vi "Attocubes_test.vi"() -> ()   [LabVIEW 2019]
panel:
  in  "Stop":bool
  out "Position [µm | m°] 2":dbl format="%.3g"
  in  "Axis IN":u8(ring) items=["1", "2", "3"]
  out "axis out":u8(ring) items=["1", "2", "3"]
  out "Position [µm | m°]":dbl format="%.3g"
  out "*(type *) &x":u8
  out "Numeric":u8
  out "PosZ":dbl
  out "PosY":dbl
  out "PosX":dbl
  out "DCLvlZ":dbl
  out "FreqZ":dbl
  out "AmpZ":dbl
  out "DCLvlY":dbl
  out "FreqY":dbl
  out "AmpY":dbl
  out "DCLvlX":dbl
  out "FreqX":dbl
  out "AmpX":dbl
  out "additional features":T1
  out "features":u32 format="%08b"
  out "error ANC350v4_Dis/Connect 2":errorcluster
  out "error ANC350v4_discover":errorcluster
  out "output cluster":T2 {"DeviceType" items=["ANC350res", "ANC350num", "ANC350fps", "No device / invalid"]; "ID" format="%x"}
  out "error ANC350v4_Dis/Connect":errorcluster
  out "ANC350v4 found":u32
  out "ANC350_Handle":u64
  out "ourDLL":path
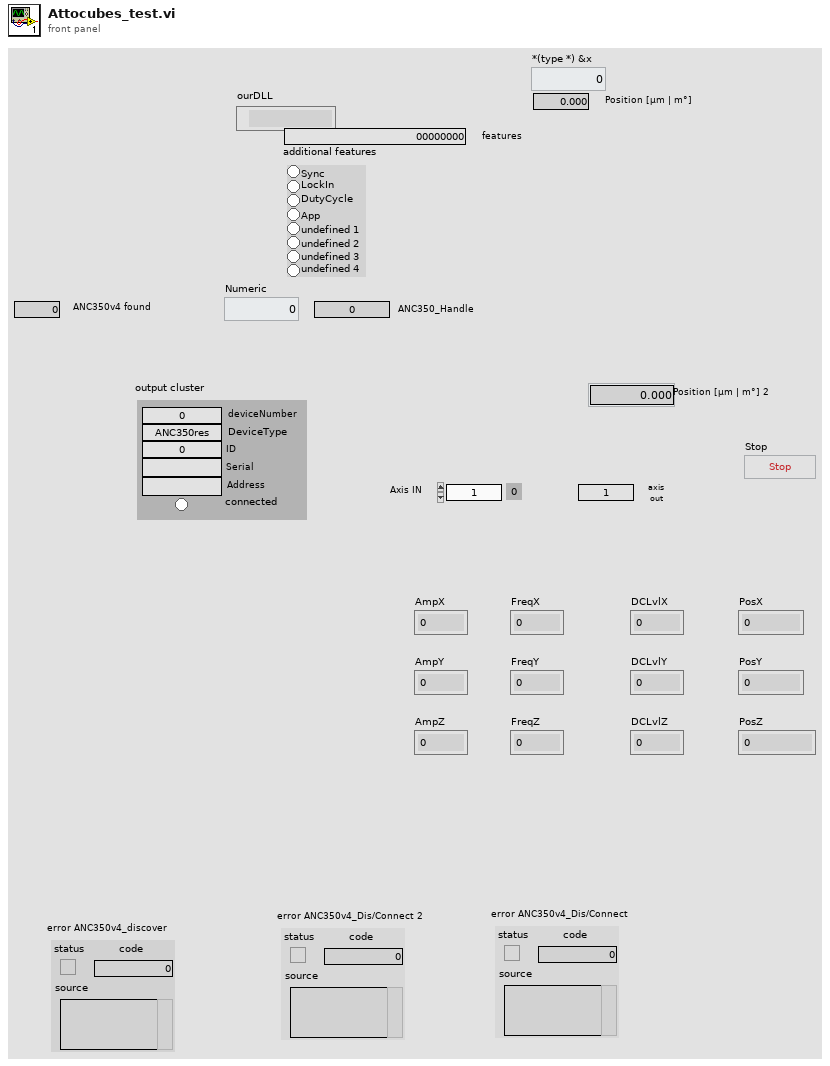
[diagram p1: front panel]
types:
  T1 = cluster{"Sync":bool, "LockIn":bool, "DutyCycle":bool, "App":bool, "undefined 1":bool, "undefined 2":bool, "undefined 3":bool, "undefined 4":bool, "undefined 7":bool}
  T2 = cluster{"deviceNumber":i32, "DeviceType":i32, "ID":u32, "Serial":string, "Address":string, "connected":bool}
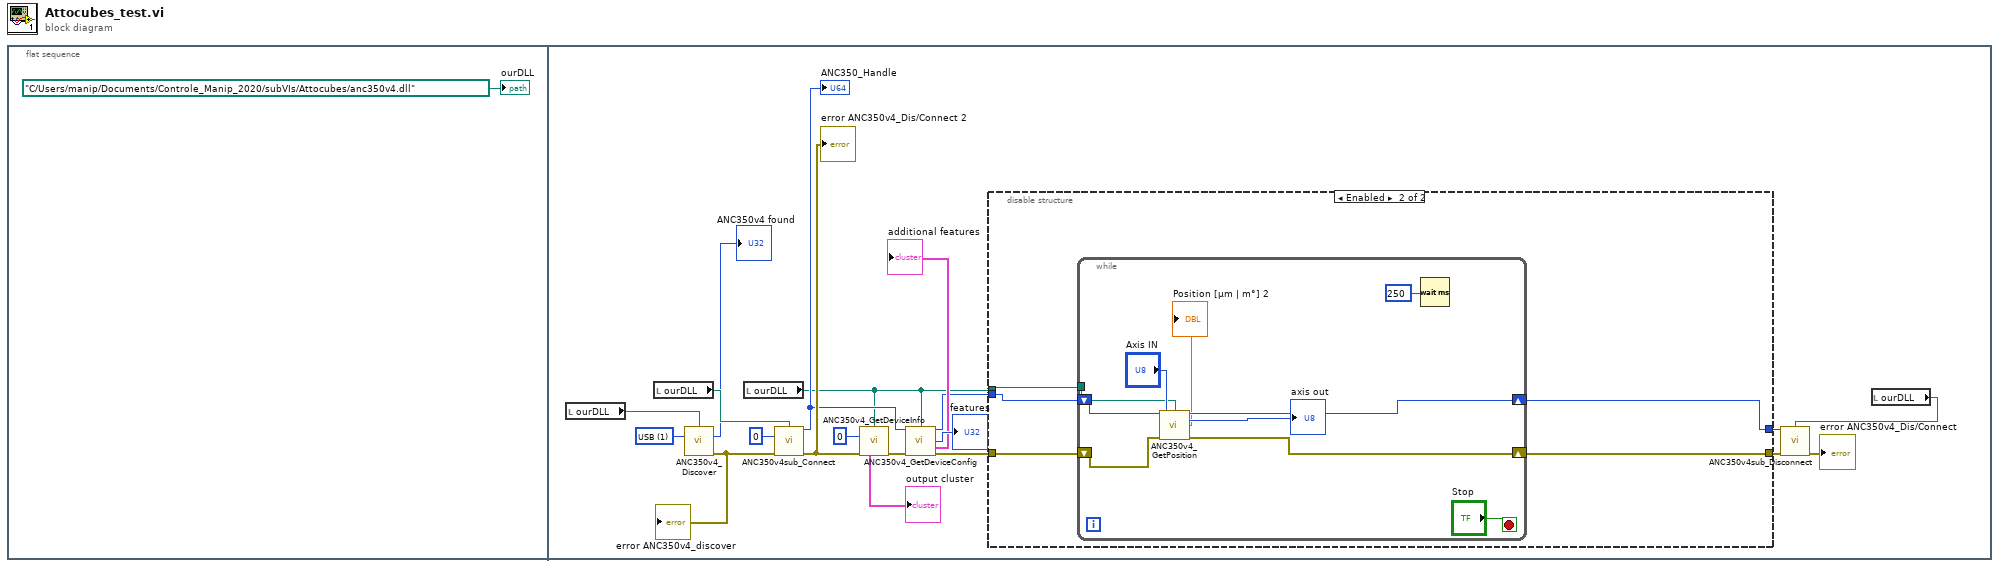
[diagram p0: block diagram]
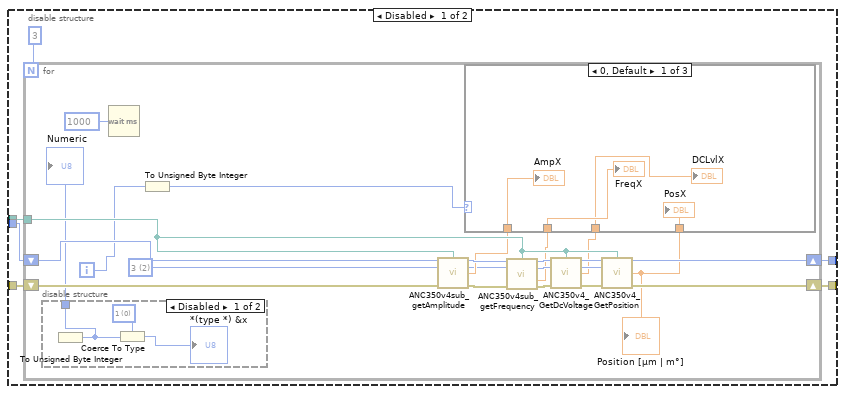
[diagram p2: hidden frame]
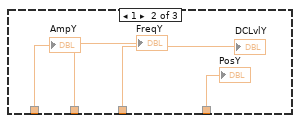
[diagram p4: hidden frame]
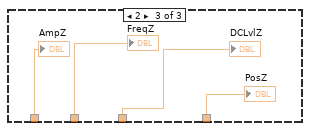
[diagram p5: hidden frame]
diagram:
  n1 = flat-sequence {
    frame #0 {
      "ourDLL" <- path "C:/Users/manip/Documents/Controle_Manip_2020/subVIs/Attocubes/anc350v4.dll"
    }
    frame #1 {
      w21 = u32 1 items=["None", "USB", "TCP", "All"] ("Interface types")
      n2 = local read "ourDLL"() -> (w14:path)
      n3 = local read "ourDLL"() -> (w20:path)
      n4 = call "ANC350v4_Discover.vi"("Path to *.DLL"=w14, "Interface types"=w21) -> ("ANC350v4 found"=→"ANC350v4 found":u32, "error ANC350v4_discover"=w19:errorcluster)  [unwired: 12 in]
      "error ANC350v4_discover" <- w19
      n5 = local read "ourDLL"() -> (w7:path)
      n6 = call "ANC350v4sub_Connect.vi"("Path to *.DLL"=w20, "deviceNumber"=0, "error in"=w19) -> ("ANC350v4_Handle_Out"=w11:u64, "error ANC350v4_Dis/Connect"=w15:errorcluster)  [unwired: 11 in]
      "ANC350_Handle" <- w11
      "error ANC350v4_Dis/Connect 2" <- w15
      n7 = call "ANC350v4_GetDeviceInfo.vi"("Path to *.DLL"=w7, "deviceNumber"=u32 0, "error in"=w15) -> ("output cluster"=→"output cluster":T2, "Error_ANC350v4_getDeviceInfo"=w10:errorcluster)  [unwired: 5 in, 6 out]
      n8 = call "ANC350v4_GetDeviceConfig.vi"("deviceHandle"=w11, "Path to *.DLL"=w7, "error in"=w10) -> ("deviceHandle"=w6:u64, "features"=→"features":u32, "additional features"=→"additional features":T1, "Error_ANC350v4_getDeviceConfig"=w4:errorcluster)  [unwired: 9 in]
      n9 = disable-structure shown="Enabled" {
        disable-tunnel: w7 -> [w27 w66]
        disable-tunnel: w6 -> [w26 w70]
        disable-tunnel: [w25 w68] -> w5
        disable-tunnel: w4 -> [w24 w69]
        disable-tunnel: [w23 w67] -> w3
        frame Disabled {
          n10 = for {
            N: 3 -> [_]
            tunnel: w27 -> [w42]
            shift-right: [w40] -> w25
            shift-left: w24 -> [w39]
            shift-right: [w38] -> w23
            shift-left: w26 -> [w41]
            i -> [w29]
            w28 = u8 2 items=["1", "2", "3"] ("axis")
            n11 = disable-structure shown="Disabled" {
              disable-tunnel: [w51 _] -> w31
              frame Disabled {
                w53 = u8 0 items=["1", "2", "3"] ("axis")
                n12 = To Unsigned Byte Integer() -> (unsigned 8bit integer=w51:u8)  [unwired: 1 in]
                n13 = Coerce To Type(0:w51, 1:w53) -> (2:→"*(type *) &x":u8)
              }
              frame Enabled {
              }
            }
            "Numeric" <- w31
            n14 = Wait (ms)(milliseconds to wait=u32 1000) -> ()  [unwired: 1 out]
            n15 = To Unsigned Byte Integer(number=w29) -> (unsigned 8bit integer=w30:u8)
            n16 = call "ANC350v4sub_getAmplitude.vi"("deviceHandle"=w41, "Path to *.DLL"=w42, "axis"=w28, "error in"=w39) -> ("deviceHandle"=w43:u64, "axis"=w32:u8, "amplitude out"=w37:dbl, "error ANC350v4_Amplitude"=w44:errorcluster)  [unwired: 8 in]
            n17 = call "ANC350v4sub_getFrequency.vi"("deviceHandle"=w43, "Path to *.DLL"=w42, "axis"=w32, "error in"=w44) -> ("deviceHandle"=w47:u64, "axis"=w46:u8, "Frequency [Hz] out"=w36:dbl, "error ANC350v4_frequency"=w45:errorcluster)  [unwired: 8 in]
            n18 = call "ANC350v4_GetDcVoltage.vi"("deviceHandle"=w47, "Path to *.DLL"=w42, "axis"=w46, "error in"=w45) -> ("deviceHandle"=w50:u64, "axis"=w49:u8, "voltage"=w35:dbl, "error ANC350v4_getDcVoltage"=w48:errorcluster)  [unwired: 8 in]
            n19 = call "ANC350v4_GetPosition.vi"("deviceHandle"=w50, "Path to *.DLL"=w42, "axis"=w49, "error in"=w48) -> ("deviceHandle"=w38:u64, "Position [µm | m°]"=w34:dbl, "error ANC350v4_getPosition"=w40:errorcluster)  [unwired: 8 in, 1 out]
            "Position [µm | m°]" <- w34
            n20 = case shown="0, Default" w30 {
              tunnel: w37 -> [w57 w61 w65]
              tunnel: w36 -> [w56 w60 w64]
              tunnel: w35 -> [w55 w59 w63]
              tunnel: w34 -> [w54 w58 w62]
              frame 0, Default {
                "FreqX" <- w56
                "AmpX" <- w57
                "DCLvlX" <- w55
                "PosX" <- w54
              }
              frame 1 {
                "FreqY" <- w60
                "DCLvlY" <- w59
                "AmpY" <- w61
                "PosY" <- w58
              }
              frame 2 {
                "FreqZ" <- w64
                "DCLvlZ" <- w63
                "AmpZ" <- w65
                "PosZ" <- w62
              }
            }
          }
        }
        frame Enabled {
          n21 = while {
            tunnel: w66 -> [w74]
            shift-right: [w77] -> w67
            shift-left: w70 -> [w80]
            shift-right: [w78] -> w68
            shift-left: w69 -> [w79]
            stop <- "Stop" stop-if-true
            n22 = call "ANC350v4_GetPosition.vi"("deviceHandle"=w80, "Path to *.DLL"=w74, "axis"="Axis IN", "error in"=w79) -> ("deviceHandle"=w77:u64, "axis"=→"axis out":u8, "Position [µm | m°]"=→"Position [µm | m°] 2":dbl, "error ANC350v4_getPosition"=w78:errorcluster)  [unwired: 8 in]
            n23 = Wait (ms)(milliseconds to wait=u32 250) -> ()  [unwired: 1 out]
          }
        }
      }
      n24 = local read "ourDLL"() -> (w2:path)
      n25 = call "ANC350v4sub_Disconnect.vi"("ANC350v4_Handle"=w3, "Path to *.DLL"=w2, "error in"=w5) -> ("error ANC350v4_Dis/Connect"=→"error ANC350v4_Dis/Connect":errorcluster)  [unwired: 12 in]
    }
  }
